vi "p31transformaciones.vi"() -> ()   [LabVIEW 2017]
panel:
  in  "escala":dbl(slide) scale=0.0..3.0
  in  "rotar":dbl(knob) scale=0.0..360.0
  in  "Y":dbl(slide) scale=-500.0..500.0
  in  "X":dbl(slide) scale=-500.0..500.0
  out "new picture 2":picture
  out "new picture":picture
  in  "path to BMP file":path
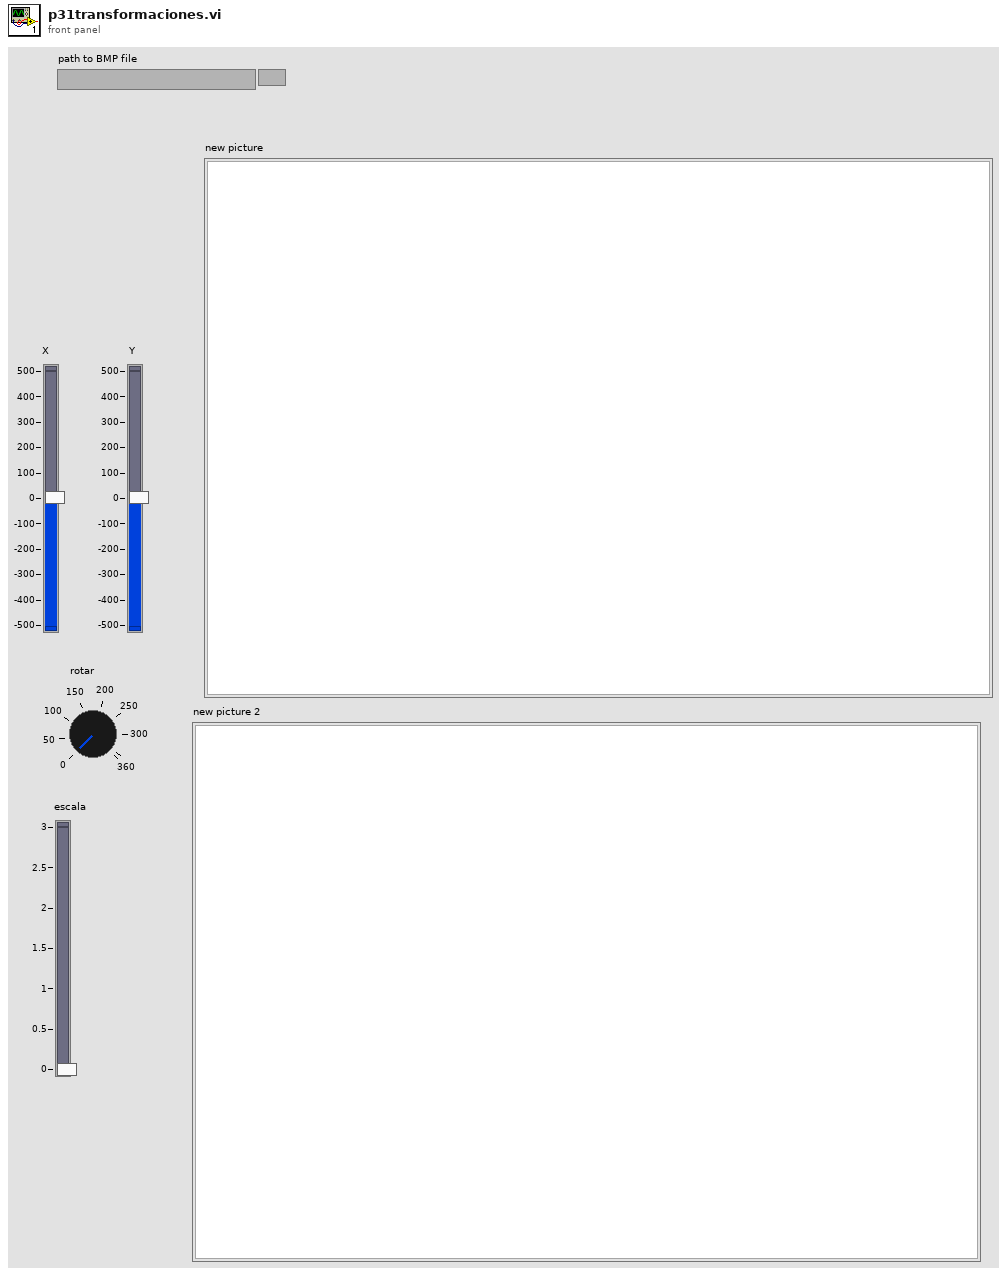
[diagram p1: front panel]
types:
  T1 = typedef "imagedata.ctl" = cluster{"image type":i32, "image depth":i32, "image":u8[], "mask":u8[], "colors":u32[], "Rectangle":cluster{"left":i16, "top":i16, "right":i16, "bottom":i16}}
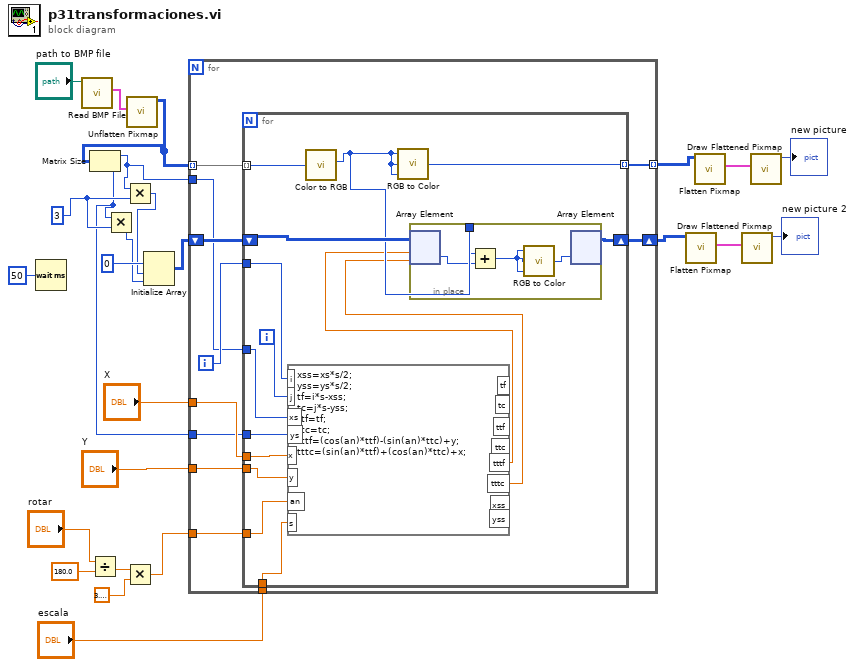
[diagram p0: block diagram]
diagram:
  w5 = 3
  n1 = Wait (ms)(milliseconds to wait=u32 50) -> ()  [unwired: 1 out]
  n2 = call <vilib>:"Read BMP File.vi"("path to BMP file"="path to BMP file") -> ("image data"=w23:T1)  [unwired: 8 in, 2 out]
  n3 = Divide(x="rotar", y=180.0) -> (x/y=w10:dbl)
  n4 = Multiply(x=w10, y=3.141592653589793) -> (x*y=w8:dbl)
  n5 = call <vilib>:"Unflatten Pixmap.vi"("image data"=w23) -> ("24-bit pixmap"=w20:u32[][])  [unwired: 4 in, 6 out]
  n6 = Matrix Size(0:w20) -> (1:w2:i32, 2:w1:i32)
  n7 = Multiply(x=w1, y=w5) -> (x*y=w3:i32)
  n8 = Multiply(x=w2, y=w5) -> (x*y=w4:i32)
  n9 = Initialize Array(0, w4, w3) -> (w19:i32[][])
  n10 = for {
    tunnel: w20 -> [w36] mode=indexing
    tunnel: [w35] -> w22 mode=indexing
    shift-right: [w32] -> w15
    shift-left: w19 -> [w34]
    tunnel: "X" -> [w31]
    tunnel: "Y" -> [w30]
    tunnel: w8 -> [w29]
    tunnel: "escala" -> [w28]
    tunnel: w2 -> [w27]
    tunnel: w1 -> [w26]
    i -> [w33]
    n11 = for {
      tunnel: w36 -> [w51] mode=indexing
      tunnel: [w50] -> w35 mode=indexing
      tunnel: w33 -> [w46]
      shift-right: [w47] -> w32
      shift-left: w34 -> [w49]
      tunnel: w31 -> [w44]
      tunnel: w30 -> [w43]
      tunnel: w29 -> [w42]
      tunnel: w28 -> [w41]
      tunnel: w27 -> [w38]
      tunnel: w26 -> [w37]
      i -> [w45]
      n12 = formula code="xss=xs*s/2;\nyss=ys*s/2;\ntf=i*s-xss;\ntc=j*s-yss;\nttf=tf;\nttc=tc;\ntttf=(cos(an)*ttf)-(sin(an)*ttc)+y;\ntttc=(sin(an)*ttf)+(cos(an)*ttc)+x;"("i"=w46, "j"=w45, "x"=w44, "y"=w43, "an"=w42, "s"=w41, "xs"=w38, "ys"=w37) -> ("tttf"=w40:dbl, "tttc"=w39:dbl)  [unwired: 6 out]
      n13 = call <vilib>:"Color to RGB.vi"("Color"=w51) -> ("R"=w48:u8)  [unwired: 3 out]
      n14 = call <vilib>:"RGB to Color.vi"("B"=w48, "G"=w48, "R"=w48) -> ("Color"=w50:u32)
      n15 = in-place {
        in-place-border: w48 -> [w55]
        n16 = in-place-array #1(w49, w40, w39) -> (w54:i32)
        n17 = Add(x=w55, y=w54) -> (x+y=w53:i32)
        n18 = call <vilib>:"RGB to Color.vi"("B"=w53, "G"=w53, "R"=w53) -> ("Color"=w52:u32)
        n19 = in-place-array #1(w52) -> (w47:i32[][])  [unwired: 2 out]
      }
    }
  }
  n20 = call <vilib>:"Flatten Pixmap.vi"("24-bit pixmap"=w15) -> ("image data"=w17:T1)  [unwired: 10 in]
  n21 = call <vilib>:"Flatten Pixmap.vi"("24-bit pixmap"=w22) -> ("image data"=w21:T1)  [unwired: 10 in]
  n22 = call <vilib>:"Draw Flattened Pixmap.vi"("image data"=w17) -> ("new picture"=→"new picture 2":picture)  [unwired: 8 in]
  n23 = call <vilib>:"Draw Flattened Pixmap.vi"("image data"=w21) -> ("new picture"=→"new picture":picture)  [unwired: 8 in]
